vi "Benchmarking Asynchronous Calls.vi"() -> ()   [LabVIEW 2019]
doc: "This example requests web pages from the specified servers using an HTTP Get request and records how long the requests take. This example demonstrates and compares four different design patterns that accomplish this task:\n\n* Call By Reference node inside a For Loop to sequentially call the target VI\n* Call By Reference node inside a Parallel For Loop to allow some calls to execute in parallel depending on the number of CPU cores\n* Run VI method to execute all calls in parallel\n* Asynchronously calling VIs using the Start Asynchronous Call node to execute all calls in parallel\n\nIn general, if an application is I/O bound (ex: communication over the network), the parallel call approaches perform better. The default behavior of the Parallel For loop will run frames in parallel based on the number of CPU cores. The Run VI method and asynchronous call patterns allow a user to define the amount of parallelism at run time. \n\nIf an application is local CPU bound, the Parallel For Loop approach will perform the best. It utilizes the number of CPU cores and has less overhead when compared to the Run VI method and the asynchronous call pattern.\n\nThe actual performance results for this example depend largely on the computer and network connection.\n\nThe asynchronous call pattern and the Run VI method require overhead to allow the run-time defined parallelism. This overhead is negligible when compared to the I/O usage as in this example. The asynchronous call pattern has less overhead than the Run VI method. Depending on the application, the asynchronous call pattern might require LabVIEW to open fewer VI references and is more efficient when passing parameters to and from the target VI. The asynchronous call pattern also has a simpler syntax than the Run VI method."
panel:
  in  "Address":string="Address"
  out "Progress 3":i32(slide) scale=0.0..8.0
  out "Progress 2":i32(slide) scale=0.0..8.0
  out "Progress 1":i32(slide) scale=0.0..8.0
  out "Progress 0":i32(slide) scale=0.0..8.0
  out "Asynchronous Call By Reference":dbl
  out "Run VI Method":dbl
  out "Call By Reference (Parallel For Loop)":dbl
  out "Call By Reference":dbl
  # "Overview: Demonstrates the performance of Asynchronous VI Calls against other VI calling techniques.\nRequirements: A network connection\nInstructions:\nRun the VI. Observe the benchmark values below. Note that these times may be affected by network issues. See the block diagram for more information."
  # "Note: In general, if an application is I/O bound (communication over the network, e.g.), the parallel call approaches perform better. The default behavior of the Parallel For Loop will run frames in parallel based on the number of CPU cores. The Run VI method and asynchronous call patterns allow a user to define the amount of parallelism at run time. If an application is local CPU bound, the Parallel For Loop approach will perform the best. It utilizes the number of CPU cores and has less overhead when compared to the Run VI method and the asynchronous call pattern.\n\nThe asynchronous call pattern and the Run VI method require overhead to allow the run-time defined parallelism. This overhead is negligible when compared to the I/O usage as in this example. The asynchronous call pattern has less overhead than the Run VI method. Depending on the application, the asynchronous call pattern might require LabVIEW to open fewer VI references and is more efficient when passing parameters to and from the target VI. The asynchronous call pattern also has a simpler syntax than the Run VI method."
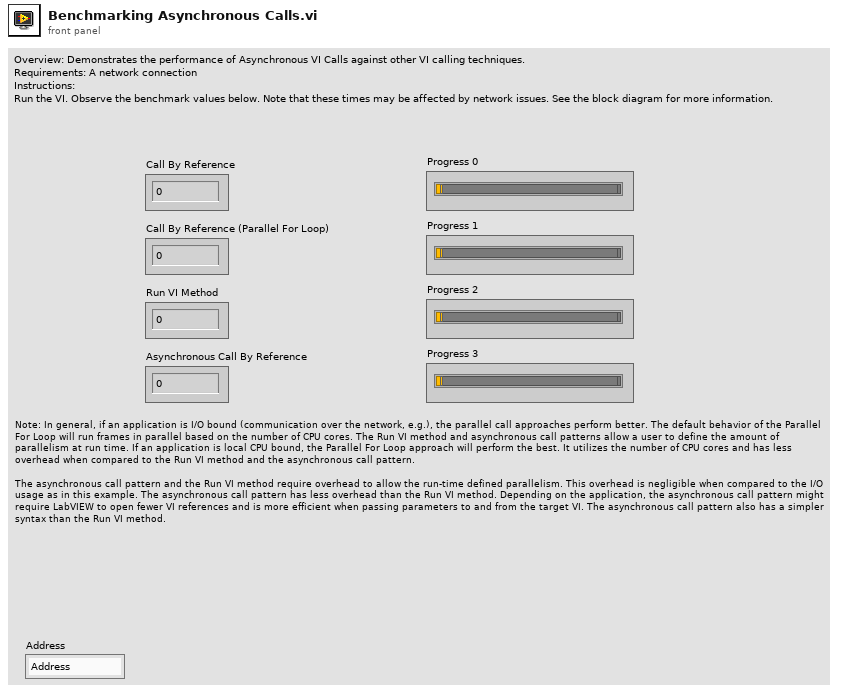
[diagram p1: front panel]
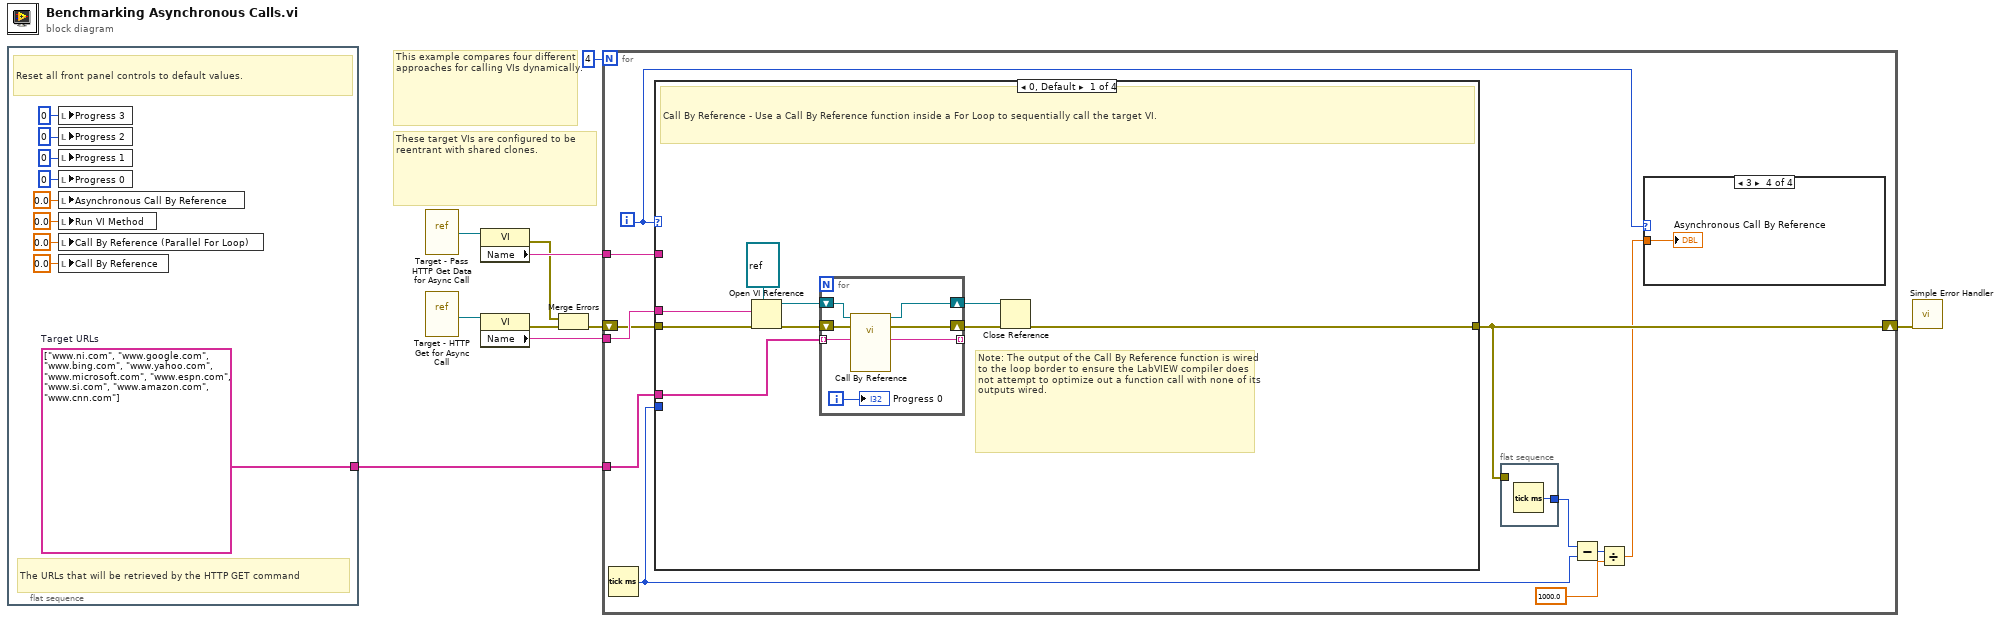
[diagram p0: block diagram]
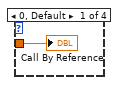
[diagram p2: hidden frame]
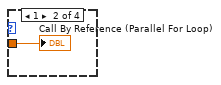
[diagram p3: hidden frame]
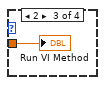
[diagram p4: hidden frame]
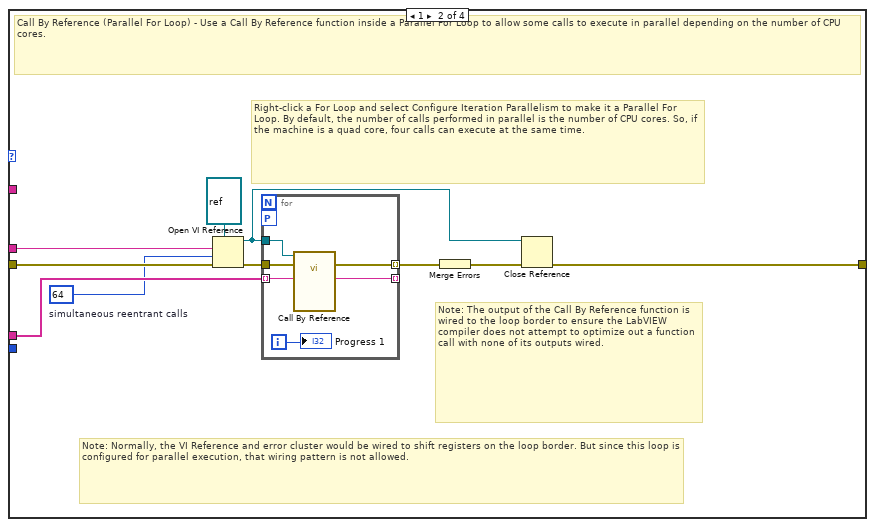
[diagram p5: hidden frame]
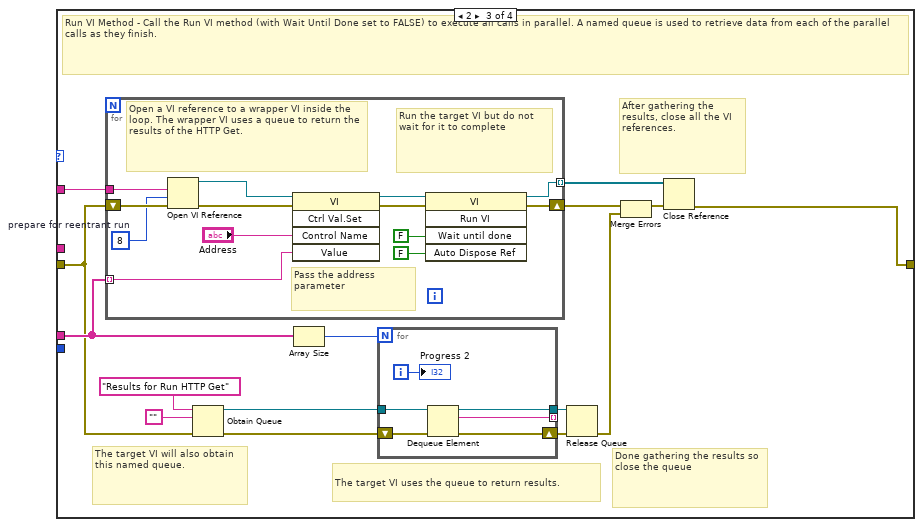
[diagram p6: hidden frame]
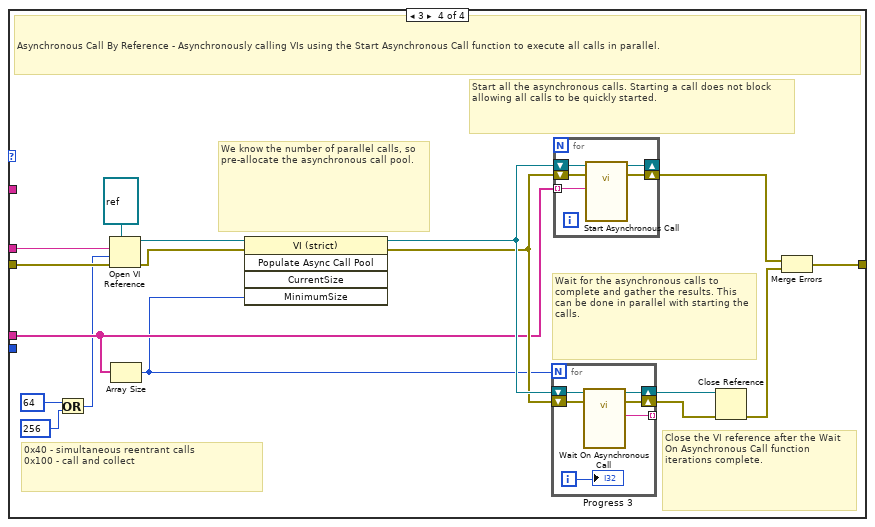
[diagram p7: hidden frame]
diagram:
  # "This example compares four different approaches for calling VIs dynamically."
  # "These target VIs are configured to be reentrant with shared clones."
  n1 = flat-sequence {
    tunnel: [w11] -> w1
    frame #0 {
      w11 = string[] ["www.ni.com", "www.google.com", "www.bing.com", "www.yahoo.com", "www.microsoft.com", "www.espn.com", "www.si.com", "www.amazon.com", "www.cnn.com"]  # Target URLs
      # "The URLs that will be retrieved by the HTTP GET command"
      # "Reset all front panel controls to default values."
      n2 = local write "Progress 3"(0 ("Progress 3")) -> ()
      n3 = local write "Progress 2"(0 ("Progress 2")) -> ()
      n4 = local write "Progress 1"(0 ("Progress 1")) -> ()
      n5 = local write "Progress 0"(0 ("Progress 0")) -> ()
      n6 = local write "Asynchronous Call By Reference"(0.0 ("Asynchronous Call By Reference")) -> ()
      n7 = local write "Run VI Method"(0.0 ("Run VI Method")) -> ()
      n8 = local write "Call By Reference (Parallel For Loop)"(0.0 ("Call By Reference (Parallel For Loop)")) -> ()
      n9 = local write "Call By Reference"(0.0 ("Call By Reference")) -> ()
    }
  }
  n10 = vi-ref "Target - Pass HTTP Get Data for Async Call.vi"() -> (w7:refnum<vi>)
  n11 = vi-ref "Target - HTTP Get for Async Call.vi"() -> (w10:refnum<vi>)
  n12 = property class="VI"(reference=w7) -> (error out=w2:errorcluster, "Name"=w6:string)  [unwired: 1 in, 1 out]
  n13 = property class="VI"(reference=w10) -> (error out=w8:errorcluster, "Name"=w9:string)  [unwired: 1 in, 1 out]
  n14 = Merge Errors(w2, w8) -> (w3:errorcluster)
  n15 = for {
    N: 4 -> [_]
    tunnel: w9 -> [w30]
    tunnel: w1 -> [w28]
    tunnel: w6 -> [w27]
    shift-right: [w26] -> w5
    shift-left: w3 -> [w29]
    i -> [w21]
    n16 = Tick Count (ms)() -> (millisecond timer value=w22:u32)
    n17 = case shown="0, Default" w21 {
      tunnel: w30 -> [w44 w61 _ w118]
      tunnel: w29 -> [w43 w60 w68 w117]
      tunnel: w28 -> [w39 w58 w70 w110]
      tunnel: w22 -> [_ _ _ _]
      tunnel: [w36 w57 w71 w107] -> w26
      tunnel: w27 -> [_ _ w82 _]
      frame 0, Default {
        # "Note: The output of the Call By Reference function is wired to the loop border to ensure the LabVIEW compiler does not attempt to optimize out a function call with none of its outputs wired."
        # "Call By Reference - Use a Call By Reference function inside a For Loop to sequentially call the target VI."
        n18 = Open VI Reference(type specifier VI Refnum (for type only)=refnum<vi> refnum, vi path=w44, error in (no error)=w43) -> (vi reference=w41:refnum<vi>, error out=w40:errorcluster)  [unwired: 3 in]
        n19 = for {
          tunnel: w39 -> [w49] mode=indexing
          shift-right: [w48] -> w38
          shift-left: w41 -> [w51]
          shift-right: [w47] -> w37
          shift-left: w40 -> [w50]
          tunnel: [w46] -> _ mode=indexing
          i -> [w45]
          n20 = call-by-ref "?"(reference=w51, error in=w50, "Address"=w49) -> (reference out=w48:refnum<vi>, error out=w47:errorcluster, "Results"=w46:string)  [unwired: 10 in]
          "Progress 0" <- w45
        }
        n21 = Close Reference(reference=w38, error in (no error)=w37) -> (error out=w36:errorcluster)
      }
      frame 1 {
        w56 = 64  # simultaneous reentrant calls
        # "Note: Normally, the VI Reference and error cluster would be wired to shift registers on the loop border. But since this loop is configured for parallel execution, that wiring pattern is not allowed."
        # "Note: The output of the Call By Reference function is wired to the loop border to ensure the LabVIEW compiler does not attempt to optimize out a function call with none of its outputs wired."
        # "Right-click a For Loop and select Configure Iteration Parallelism to make it a Parallel For Loop. By default, the number of calls performed in parallel is the number of CPU cores. So, if the machine is a quad core, four calls can execute at the same time."
        # "Call By Reference (Parallel For Loop) - Use a Call By Reference function inside a Parallel For Loop to allow some calls to execute in parallel depending on the number of CPU cores."
        n22 = Open VI Reference(type specifier VI Refnum (for type only)=refnum<vi> refnum, vi path=w61, options=w56, error in (no error)=w60) -> (vi reference=w53:refnum<vi>, error out=w55:errorcluster)  [unwired: 2 in]
        n23 = for {
          tunnel: w58 -> [w67] mode=indexing
          tunnel: [w66] -> _ mode=indexing
          workers-P: _ -> [_]
          tunnel: w53 -> [w65]
          tunnel: w55 -> [w64]
          tunnel: [w63] -> w54 mode=indexing
          i -> [w62]
          n24 = call-by-ref "?"(reference=w65, error in=w64, "Address"=w67) -> (error out=w63:errorcluster, "Results"=w66:string)  [unwired: 10 in, 1 out]
          "Progress 1" <- w62
        }
        n25 = Merge Errors(w54) -> (w52:errorcluster)
        n26 = Close Reference(reference=w53, error in (no error)=w52) -> (error out=w57:errorcluster)
      }
      frame 2 {
        # "After gathering the results, close all the VI references."
        # "Done gathering the results so close the queue"
        # "The target VI uses the queue to return results."
        # "The target VI will also obtain this named queue."
        # "Run VI Method - Call the Run VI method (with Wait Until Done set to FALSE) to execute all calls in parallel. A named queue is used to retrieve data from each of the parallel calls as they finish."
        n27 = for {
          tunnel: w82 -> [w100]
          tunnel: w70 -> [w91] mode=indexing
          tunnel: [w90] -> w73 mode=indexing
          shift-right: [w89] -> w74
          shift-left: w68 -> [w101]
          w99 = 8  # prepare for reentrant run
          # "Open a VI reference to a wrapper VI inside the loop. The wrapper VI uses a queue to return the results of the HTTP Get."
          # "Pass the address parameter"
          # "Run the target VI but do not wait for it to complete"
          n28 = Open VI Reference(vi path=w100, options=w99, error in (no error)=w101) -> (vi reference=w96:refnum<vi>, error out=w95:errorcluster)  [unwired: 3 in]
          n29 = invoke class="VI" method="Ctrl Val.Set"(reference=w96, error in=w95, "Control Name"="Address", "Value"=w91) -> (reference out=w93:refnum<vi>, error out=w92:errorcluster)  [unwired: 1 in, 3 out]
          n30 = invoke class="VI" method="Run VI"(reference=w93, error in=w92, "Wait until done"=FALSE ("Wait Until Done"), "Auto Dispose Ref"=FALSE ("Auto Dispose Reference")) -> (reference out=w90:refnum<vi>, error out=w89:errorcluster)  [unwired: 1 in, 3 out]
        }
        n31 = Obtain Queue(name (unnamed)="Results for Run HTTP Get", element data type="", error in (no error)=w68) -> (queue out=w79:refnum<queue>, error out=w78:errorcluster)  [unwired: 2 in, 1 out]
        n32 = Array Size(array=w70) -> (size(s)=w69:i32)
        n33 = for {
          N: w69 -> [_]
          tunnel: w79 -> [w88]
          shift-right: [w84] -> w76
          shift-left: w78 -> [w87]
          tunnel: [w85] -> w77
          tunnel: [w86] -> _ mode=indexing
          i -> [w83]
          n34 = Dequeue Element(queue=w88, error in (no error)=w87) -> (queue out=w85:refnum<queue>, element=w86:string, error out=w84:errorcluster)  [unwired: 1 in, 1 out]
          "Progress 2" <- w83
        }
        n35 = Release Queue(queue=w77, error in (no error)=w76) -> (error out=w75:errorcluster)  [unwired: 1 in, 2 out]
        n36 = Merge Errors(w74, w75) -> (w72:errorcluster)
        n37 = Close Reference(reference=w73, error in (no error)=w72) -> (error out=w71:errorcluster)
      }
      frame 3 {
        # "Close the VI reference after the Wait On Asynchronous Call function iterations complete."
        # "Start all the asynchronous calls. Starting a call does not block allowing all calls to be quickly started."
        # "Wait for the asynchronous calls to complete and gather the results. This can be done in parallel with starting the calls."
        # "0x40 - simultaneous reentrant calls\n0x100 - call and collect"
        # "We know the number of parallel calls, so pre-allocate the asynchronous call pool."
        # "Asynchronous Call By Reference - Asynchronously calling VIs using the Start Asynchronous Call function to execute all calls in parallel."
        n38 = Or(x=64 ("options"), y=256 ("options")) -> (x .or. y?=w102:i32)
        n39 = Open VI Reference(type specifier VI Refnum (for type only)=refnum<vi> refnum, vi path=w118, options=w102, error in (no error)=w117) -> (vi reference=w114:refnum<vi>, error out=w113:errorcluster)  [unwired: 2 in]
        n40 = Array Size(array=w110) -> (size(s)=w105:i32)
        n41 = invoke class="VI (strict)" method="Populate Async Call Pool"(reference=w114, error in=w113, "MinimumSize"=w105) -> (reference out=w112:refnum<vi>, error out=w111:errorcluster)  [unwired: 2 in, 3 out]
        n42 = for {
          N: w105 -> [_]
          shift-right: [w122] -> w115
          shift-left: w112 -> [w124]
          shift-right: [w121] -> w106
          shift-left: w111 -> [w123]
          tunnel: [w119] -> _ mode=indexing
          i -> [w120]
          n43 = call-by-ref "Wait On Asynchronous Call"(reference=w124, error in=w123) -> (reference out=w122:refnum<vi>, error out=w121:errorcluster, "Results"=w119:string)  [unwired: 11 in]
          "Progress 3" <- w120
        }
        n44 = for {
          tunnel: w110 -> [w127] mode=indexing
          shift-right: [w128] -> w109
          shift-left: w111 -> [w129]
          shift-right: [w125] -> _
          shift-left: w112 -> [w126]
          n45 = call-by-ref "Start Asynchronous Call"(reference=w126, error in=w129, "Address"=w127) -> (reference out=w125:refnum<vi>, error out=w128:errorcluster)  [unwired: 10 in, 1 out]
        }
        n46 = Close Reference(reference=w115, error in (no error)=w106) -> (error out=w108:errorcluster)
        n47 = Merge Errors(w109, w108) -> (w107:errorcluster)
      }
    }
    n48 = flat-sequence {
      tunnel: w26 -> [_]
      tunnel: [w35] -> w23
      frame #0 {
        n49 = Tick Count (ms)() -> (millisecond timer value=w35:u32)
      }
    }
    n50 = Subtract(x=w23, y=w22) -> (x-y=w25:u32)
    n51 = Divide(x=w25, y=1000.0) -> (x/y=w20:dbl)
    n52 = case shown="3" w21 {
      tunnel: w20 -> [w31 w32 w33 w34]
      frame 0, Default {
        "Call By Reference" <- w31
      }
      frame 1 {
        "Call By Reference (Parallel For Loop)" <- w32
      }
      frame 2 {
        "Run VI Method" <- w33
      }
      frame 3 {
        "Asynchronous Call By Reference" <- w34
      }
    }
  }
  n53 = call <vilib>:"Simple Error Handler.vi"("error in (no error)"=w5) -> ()  [unwired: 4 in, 5 out]
